vi "Test New Report is Opened on Seconde Test Start.vi"(8 "error in (no error)":errorcluster, 11 "XML Report Test in":refnum<class "Report Generator Test.lvclass">) -> (0 "error out":errorcluster, 3 "XML Report Test out":refnum<class "Report Generator Test.lvclass">)   [LabVIEW 2020, in "Report Generator Test.lvclass"]
uses:
  Report Generator Test.lvclass
  Report Generator Test.lvclass/Report Generator Test.ctl
  Test Doubles/Mock Report/Mock Report.lvclass
  <vilib>/Astemes/LUnit/Test Case.lvclass
  C:/Program Files (x86)/National Instruments/LabVIEW 2020/vi.lib/Astemes/LUnit/Test Case.lvclass
  C:/git/astemes-lunit/tests/Report Test/Report Generator Test.lvclass
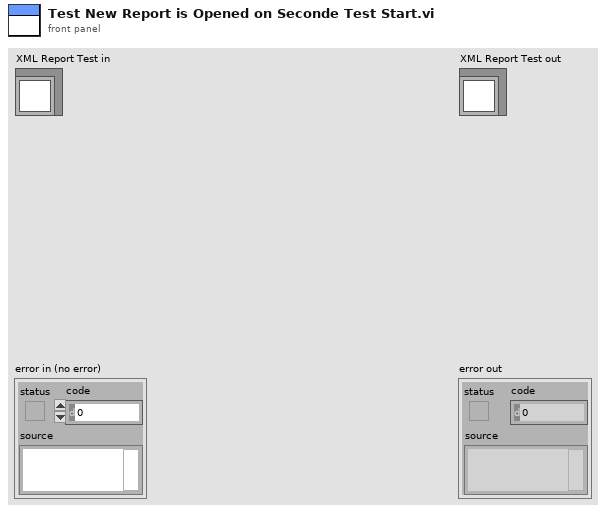
[diagram p1: front panel]
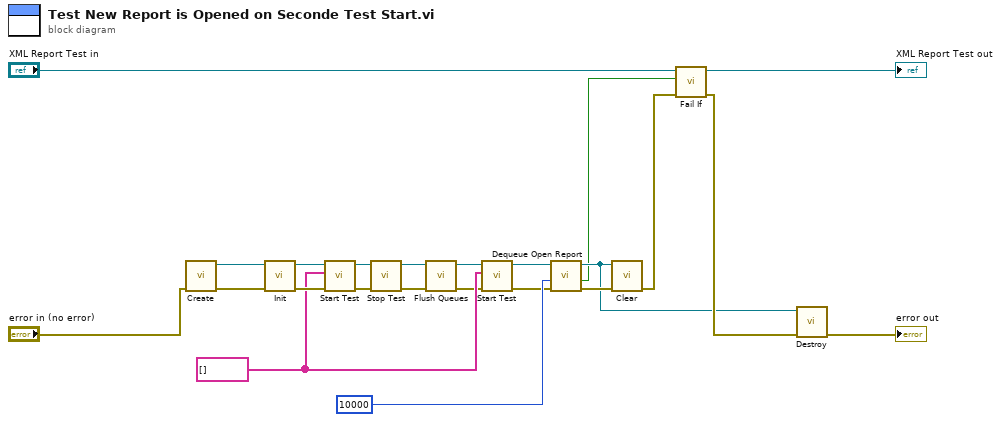
[diagram p0: block diagram]
diagram:
  w4 = string[] [] ("Tests")
  n1 = call "Create.vi"("error in (no error)"="error in (no error)") -> ("error out"=w13:errorcluster, "Mock Report Out"=w15:refnum<class "Mock Report.lvclass">)  [unwired: 9 in]
  n2 = call-dynamic "Init.vi"("error in (no error)"=w13, "Mock Report In"=w15) -> ("error out"=w19:errorcluster, "Mock Report Out"=w20:refnum<class "Mock Report.lvclass">)  [unwired: 8 in]
  n3 = call-dynamic "Start Test.vi"("error in (no error)"=w19, "Tests"=w4, "XML Report in"=w20) -> ("error out"=w18:errorcluster, "XML Report out"=w7:refnum<class "Mock Report.lvclass">)  [unwired: 7 in]
  n4 = call-dynamic "Stop Test.vi"("error in (no error)"=w18, "XML Report in"=w7) -> ("error out"=w8:errorcluster, "XML Report out"=w2:refnum<class "Mock Report.lvclass">)  [unwired: 8 in]
  n5 = call "Flush Queues.vi"("error in (no error)"=w8, "Mock Report in"=w2) -> ("error out"=w3:errorcluster, "Mock Report out"=w1:refnum<class "Mock Report.lvclass">)  [unwired: 8 in]
  n6 = call-dynamic "Start Test.vi"("error in (no error)"=w3, "Tests"=w4, "XML Report in"=w1) -> ("error out"=w6:errorcluster, "XML Report out"=w5:refnum<class "Mock Report.lvclass">)  [unwired: 7 in]
  n7 = call "Dequeue Open Report.vi"("error in (no error)"=w6, "timeout in ms (0)"=10000, "Mock Report In"=w5) -> ("error out"=w17:errorcluster, "timed out?"=w9:bool, "Mock Report Out"=w11:refnum<class "Mock Report.lvclass">)  [unwired: 5 in, 1 out]
  n8 = call-dynamic "Clear.vi"("error in (no error)"=w17, "XML Report in"=w11) -> ("error out"=w16:errorcluster)  [unwired: 9 in]
  n9 = call <vilib>:"Fail If.vi"("error in (no error)"=w16, "Fail?"=w9, "LUnit Test Case In"="XML Report Test in") -> ("error out"=w21:errorcluster, "LUnit Test Case Out"=→"XML Report Test out":refnum<class "Report Generator Test.lvclass">)  [unwired: 7 in]
  n10 = call "Destroy.vi"("error in (no error)"=w21, "Mock Report In"=w11) -> ("error out"=→"error out":errorcluster)  [unwired: 9 in]
